vi "Register by Name.vi"(7 "Event":refnum<class "Event.lvclass">, 8 "error in (no error)":errorcluster, 9 "Event Fire Handler":refnum<class "Abstract Event Message for View.lvclass">, 10 "View Name":string, 11 "Controller Actor in":refnum<class "Controller Actor.lvclass">) -> (0 "error out":errorcluster, 3 "Controller Actor out":refnum<class "Controller Actor.lvclass">)   [LabVIEW 2016, in "Event Actors.lvlib" / "Controller Actor.lvclass"]
uses:
  Controller Actor.lvclass
  Event/Event.lvclass
  Event Handlers/Abstract Event Message for View/Abstract Event Message for View.lvclass
  Controller Actor.lvclass/Controller Actor.ctl
  View Details.ctl
  <vilib>/ActorFramework/Message Enqueuer/Message Enqueuer.lvclass
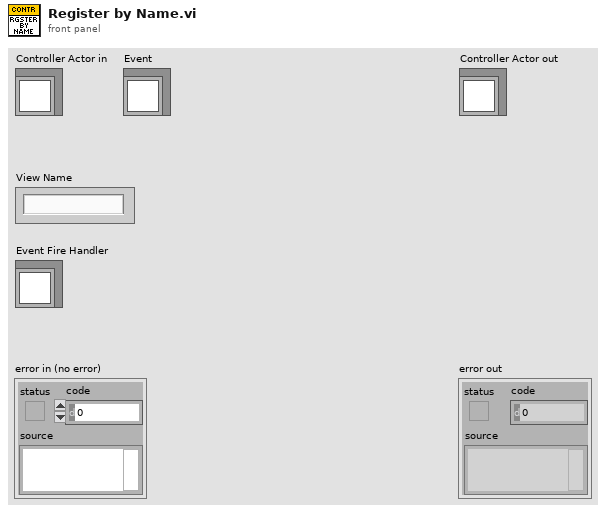
[diagram p1: front panel]
types:
  T1 = typedef "Event Actors.lvlib/Controller Actor.lvclass/View Details.ctl" = cluster{"Exclude From Broadcast":bool, "Receive Only":bool, "Paused":bool, "View Enqueuer":refnum<class "Message Enqueuer.lvclass">}
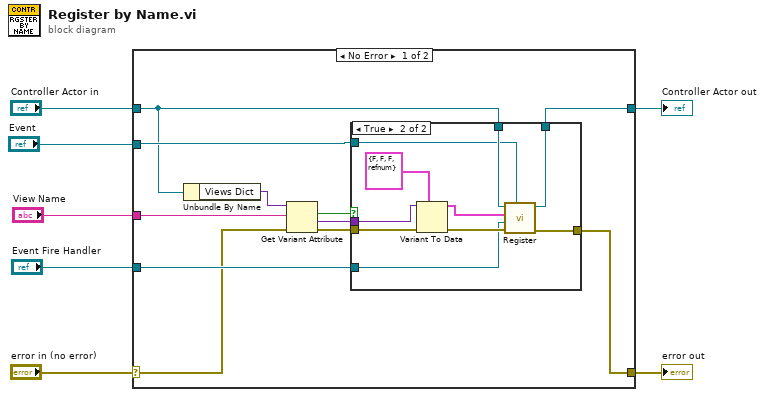
[diagram p0: block diagram]
diagram:
  n1 = case shown="No Error" "error in (no error)" {
    selector: "error in (no error)" -> [w9 w32]
    tunnel: [w8 w32] -> w6
    tunnel: [w10 w31] -> w4
    tunnel: "Controller Actor in" -> [w11 w31]
    tunnel: "View Name" -> [w17 _]
    tunnel: "Event Fire Handler" -> [w13 _]
    tunnel: "Event" -> [w12 _]
    frame No Error {
      n2 = Unbundle By Name(w11) -> ("Views Dict"=w18:variant)
      n3 = Get Variant Attribute(Variant=w18, name=w17, error in=w9) -> (found=w16:bool, value=w15:variant, error out=w14:errorcluster)  [unwired: 1 in, 1 out]
      n4 = case shown="True" w16 {
        tunnel: w15 -> [_ w29]
        tunnel: w14 -> [w20 w30]
        tunnel: w13 -> [_ w27]
        tunnel: w11 -> [w19 w26]
        tunnel: w12 -> [_ w25]
        tunnel: [w20 w24] -> w8
        tunnel: [w19 w23] -> w10
        frame False {
        }
        frame True {
          n5 = Variant To Data(error in=w30, type=T1 {"Exclude From Broadcast"=FALSE, "Receive Only"=FALSE, "Paused"=FALSE, "View Enqueuer"=refnum} ("Message Enqueuer"), Variant=w29) -> (data=w21:T1, error out=w28:errorcluster)
          n6 = call "Register.vi"("Event"=w25, "Error In"=w28, "View Event Fire Handler"=w27, "Registrant Details"=w21, "Controller Actor In"=w26) -> ("Error Out"=w24:errorcluster, "Controller Actor Out"=w23:refnum<class "Controller Actor.lvclass">)  [unwired: 5 in]
        }
      }
    }
    frame Error {
    }
  }
  "error out" <- w6
  "Controller Actor out" <- w4
